vi "GetFrameRate.vi"(8 "error in (no error)":errorcluster, 11 "CameraTestingBL in":refnum<class "CameraTesting.lvclass">) -> (0 "error out":errorcluster, 3 "CameraTestingBL out":refnum<class "CameraTesting.lvclass">)   [LabVIEW 2020, in "CameraTesting.lvlib" / "CameraTesting.lvclass"]
doc: "Get the frame rate of the camera"
uses:
  CameraTesting.lvclass
  CameraTesting.lvclass/CameraTesting.ctl
  Camera/ICamera/ICamera/ICamera.lvclass
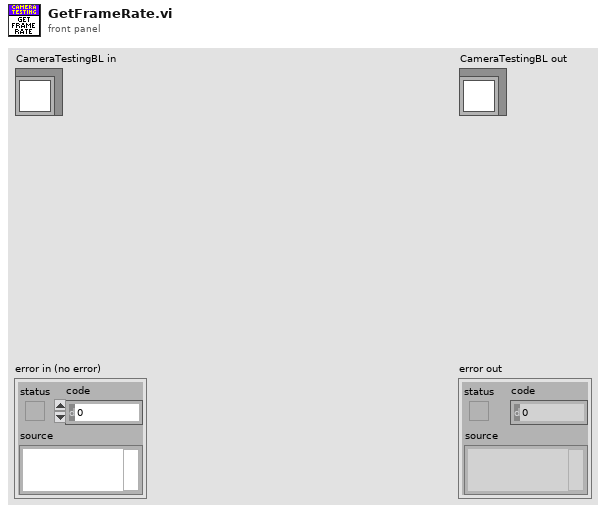
[diagram p1: front panel]
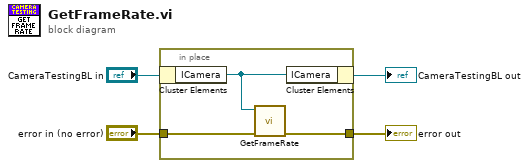
[diagram p0: block diagram]
diagram:
  n1 = in-place {
    in-place-border: "error in (no error)" -> [w7]
    in-place-border: [w6] -> w3
    n2 = in-place-cluster #1("CameraTestingBL in") -> ("ICamera"=w5:refnum<class "ICamera.lvclass">)
    n3 = call-dynamic "GetFrameRate.vi"("error in (no error)"=w7, "ICamera in"=w5) -> ("error out"=w6:errorcluster)  [unwired: 7 in, 2 out]
    n4 = in-place-cluster #1("ICamera"=w5) -> (→"CameraTestingBL out":refnum<class "CameraTesting.lvclass">)
  }
  "error out" <- w3
